vi "Measurement Logic.vi"(8 "error in":errorcluster, 9 "measurement configuration":T2={"Automation Test"=FALSE, "Power sequencing file path"="", "RFSG name"="5842_0", "RFSG port"="", "RFSG attenuation mode"=enum."Constant Attenuation", "RFSG external attenuation (dB)"=2.0, "RFSG s-parameters orientation"=enum."Port2 Towards DUT", "RFSG s2p file path"="", "RFmx name"="5842_0", "RFmx port"="", "RFmx attenuation mode"=enum."Constant Attenuation", "RFmx external attenuation (dB)"=1.2, "RFmx s-parameters orientation"=enum."Port2 Towards DUT", "RFmx s2p file path"="", "RFmx Reference Level (dBm)"=10.0, "RFSG Generation IQ Rate (S/s)"=1250000000.0, "Target Pout Per Tone (dBm)"=10.0, "Start Pin Per Tone (dBm)"=10.0, "Start Center Frequency (Hz)"=10.0, "Start Tone Spacing (Hz)"=10.0, "IM_Sweep Mode"=enum."Power", "Sweep Delay (ms)"=10, "Power Sweep End"=10.0, "Power Sweep Step"=10.0, "Frequency Sweep End"=-4.0, "Frequency Sweep Step"=1.0, "Tone Spacing Sweep End"=-4.0, "Tone Spacing Sweep Step"=1.0} {"Tone Spacing Sweep Step" format="%#.pHz"; "Tone Spacing Sweep End" format="%#.pHz"; "Frequency Sweep Step" format="%#.pHz"; "Frequency Sweep End" format="%#.pHz"; "Power Sweep End" format="%#.6f"; "Sweep Delay (ms)" format="%#_6p"; "Start Tone Spacing (Hz)" format="%#.6p"; "Start Center Frequency (Hz)" format="%#.6p"; "Start Pin Per Tone (dBm)" format="%#.6p"; "Target Pout Per Tone (dBm)" format="%#.6f"; "RFSG Generation IQ Rate (S/s)" format="%#.6f"; "RFmx Reference Level (dBm)" format="%#_6p"; "RFmx external attenuation (dB)" format="%.2f"; "RFSG external attenuation (dB)" format="%.2f"}, 10 "measure call context in":refnum<class "Measure Call Context.lvclass">) -> (0 "error out":errorcluster, 1 "measurement results":T1, 2 "measure call context out":refnum<class "Measure Call Context.lvclass">)   [LabVIEW 2023, in "FPT Intermodulation.lvclass"]
doc: "Contains the core logic for executing the measurement."
uses:
  FPT Intermodulation.lvclass
  <vilib>/Plug-In SDKs/Measurements/Measure Call Context/Measure Call Context.lvclass
  Measurement Configuration.ctl
  Measurement Results.ctl
  <extravilib>/ChannelInstances/Event Messenger-bool/Instantiate.vi
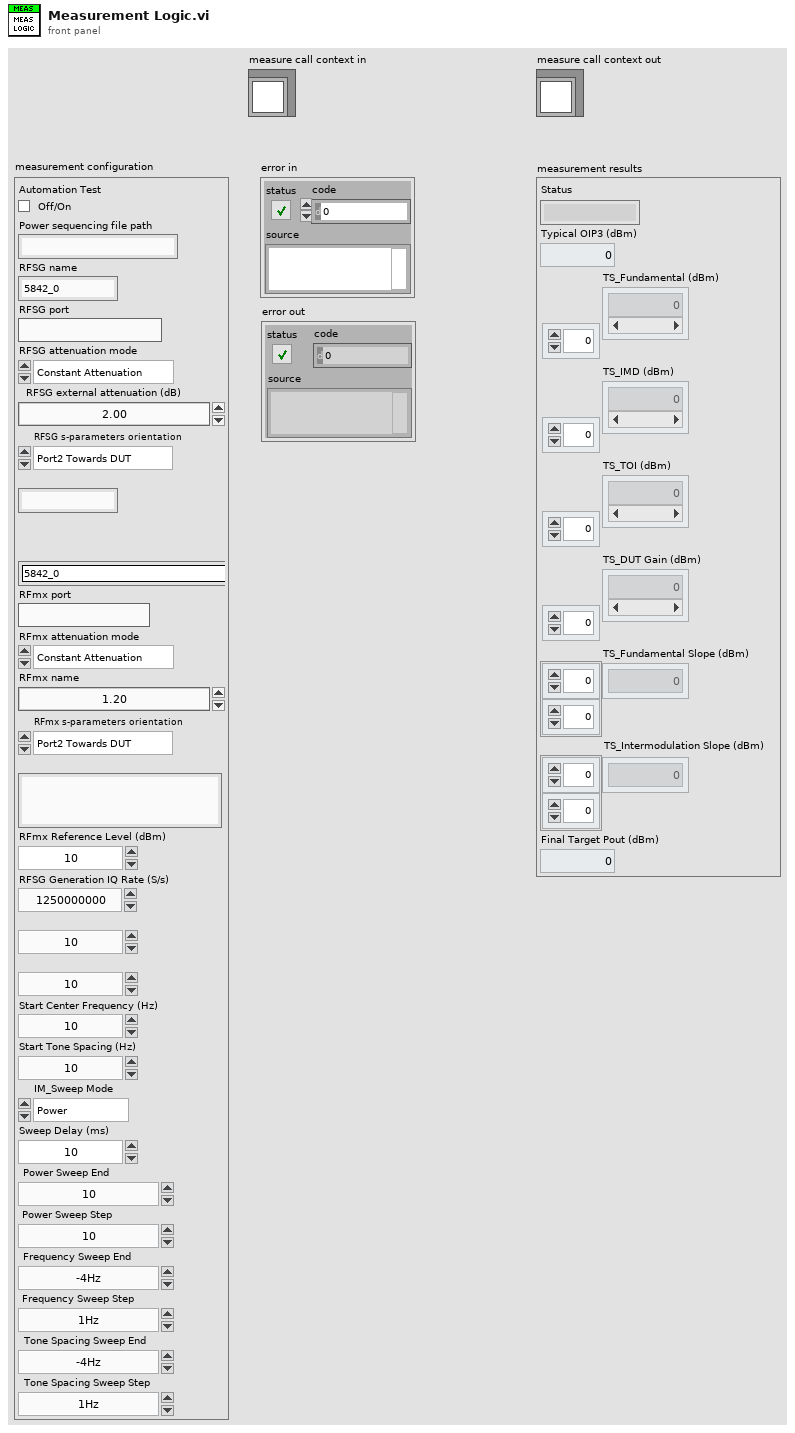
[diagram p1: front panel]
types:
  T1 = typedef "FPT Intermodulation.lvclass/Measurement Results.ctl" = cluster{"Status":string, "Typical OIP3 (dBm)":dbl, "TS_Fundamental (dBm)":dbl[][], "TS_IMD (dBm)":dbl[][], "TS_TOI (dBm)":dbl[][], "TS_DUT Gain (dBm)":dbl[][], "TS_Fundamental Slope (dBm)":dbl[][], "TS_Intermodulation Slope (dBm)":dbl[][], "Final Target Pout (dBm)":dbl}
  T2 = typedef "FPT Intermodulation.lvclass/Measurement Configuration.ctl" = cluster{"Automation Test":bool, "Power sequencing file path":string, "RFSG name":string, "RFSG port":string, "RFSG attenuation mode":enum32{"<None>", "Constant Attenuation", "s2p File"}, "RFSG external attenuation (dB)":dbl, "RFSG s-parameters orientation":enum32{"Port1 Towards DUT", "Port2 Towards DUT"}, "RFSG s2p file path":string, "RFmx name":string, "RFmx port":string, "RFmx attenuation mode":enum32{"<None>", "Constant Attenuation", "s2p File"}, "RFmx external attenuation (dB)":dbl, "RFmx s-parameters orientation":enum32{"Port1 Towards DUT", "Port2 Towards DUT"}, "RFmx s2p file path":string, "RFmx Reference Level (dBm)":dbl, "RFSG Generation IQ Rate (S/s)":dbl, "Target Pout Per Tone (dBm)":dbl, "Start Pin Per Tone (dBm)":dbl, "Start Center Frequency (Hz)":dbl, "Start Tone Spacing (Hz)":dbl, "IM_Sweep Mode":enum32{"Power", "Frequency", "Tone Spacing"}, "Sweep Delay (ms)":u32, "Power Sweep End":dbl, "Power Sweep Step":dbl, "Frequency Sweep End":dbl, "Frequency Sweep Step":dbl, "Tone Spacing Sweep End":dbl, "Tone Spacing Sweep Step":dbl}
  T3 = enum32{"Power On Dut", "De-embedding + Measurement", "Power Off Dut"}[]
  T4 = cluster{"measurement configuration":T2, "measurement results":T1}
  T5 = typedef "RFmx Config - TOI.ctl" = cluster{"Reference Level (dBm)":dbl, "Attenuation":T6}
  T6 = typedef "RFmx Config.ctl" = cluster{"RFmx Name":refnum<k15>, "RFmx Port":string, "Attenuation":cluster{"Mode":enum32{"<None>", "Constant Attenuation", "s2p File"}, "Constant Attenuation":cluster{"RFmx External Attenuation (dB)":dbl}, "s2p File":cluster{"RFmx S-Parameters Orientation":i32, "RFmx Attenuation s2p Path Name":string, "RFmx Attenuation s2p File":path}}}
  T7 = typedef "RFSG Config - TOI.ctl" = cluster{"IQ Rate (S/sec)":dbl, "Number of Samples":i32, "Attenuation":T8}
  T8 = typedef "RFsg Config.ctl" = cluster{"RFSG Name":refnum<k15>, "RFSG Port":string, "Attenuation":cluster{"Mode":enum32{"<None>", "Constant Attenuation", "s2p File"}, "Contant Attenuation":cluster{"RFSG External Attenuation (dB)":dbl}, "s2p File":cluster{"RFSG S-parameters Orientation":i32, "RFSG Attenuation s2p Path Name":string, "RFSG s2p File Path":path}}}
  T9 = typedef "Test Config - TOI.ctl" = cluster{"Target Pout Per Tone (dBm)":dbl, "Start Value":cluster{"Power Level per Tone (dBm)":dbl, "Center Frequency (Hz)":dbl, "Tone Spacing (Hz)":dbl}, "Sweep Settings":cluster{"Mode":enum16{"Power", "Frequency", "Tone Spacing"}, "Sweep Delay (ms)":u32, "Power Sweep End":dbl, "Power Sweep Step":dbl, "Frequency Sweep End":dbl, "Frequency Sweep Step":dbl, "Tone Spacing Sweep End":dbl, "Tone Spacing Sweep Step":dbl}}
  T10 = typedef "Target Pout per Tone Results Cluster - TOI.ctl" = cluster{"Target Pout per Tone (dBm)":dbl, "OIP3 (dBm)":dbl, "IIP3 (dBm)":dbl, "Pin per Tone (dBm)":dbl, "IMD (dBm)":dbl}
  T11 = typedef "Event Messenger-bool.lvlib/))Channel.ctl" = refnum<queue>
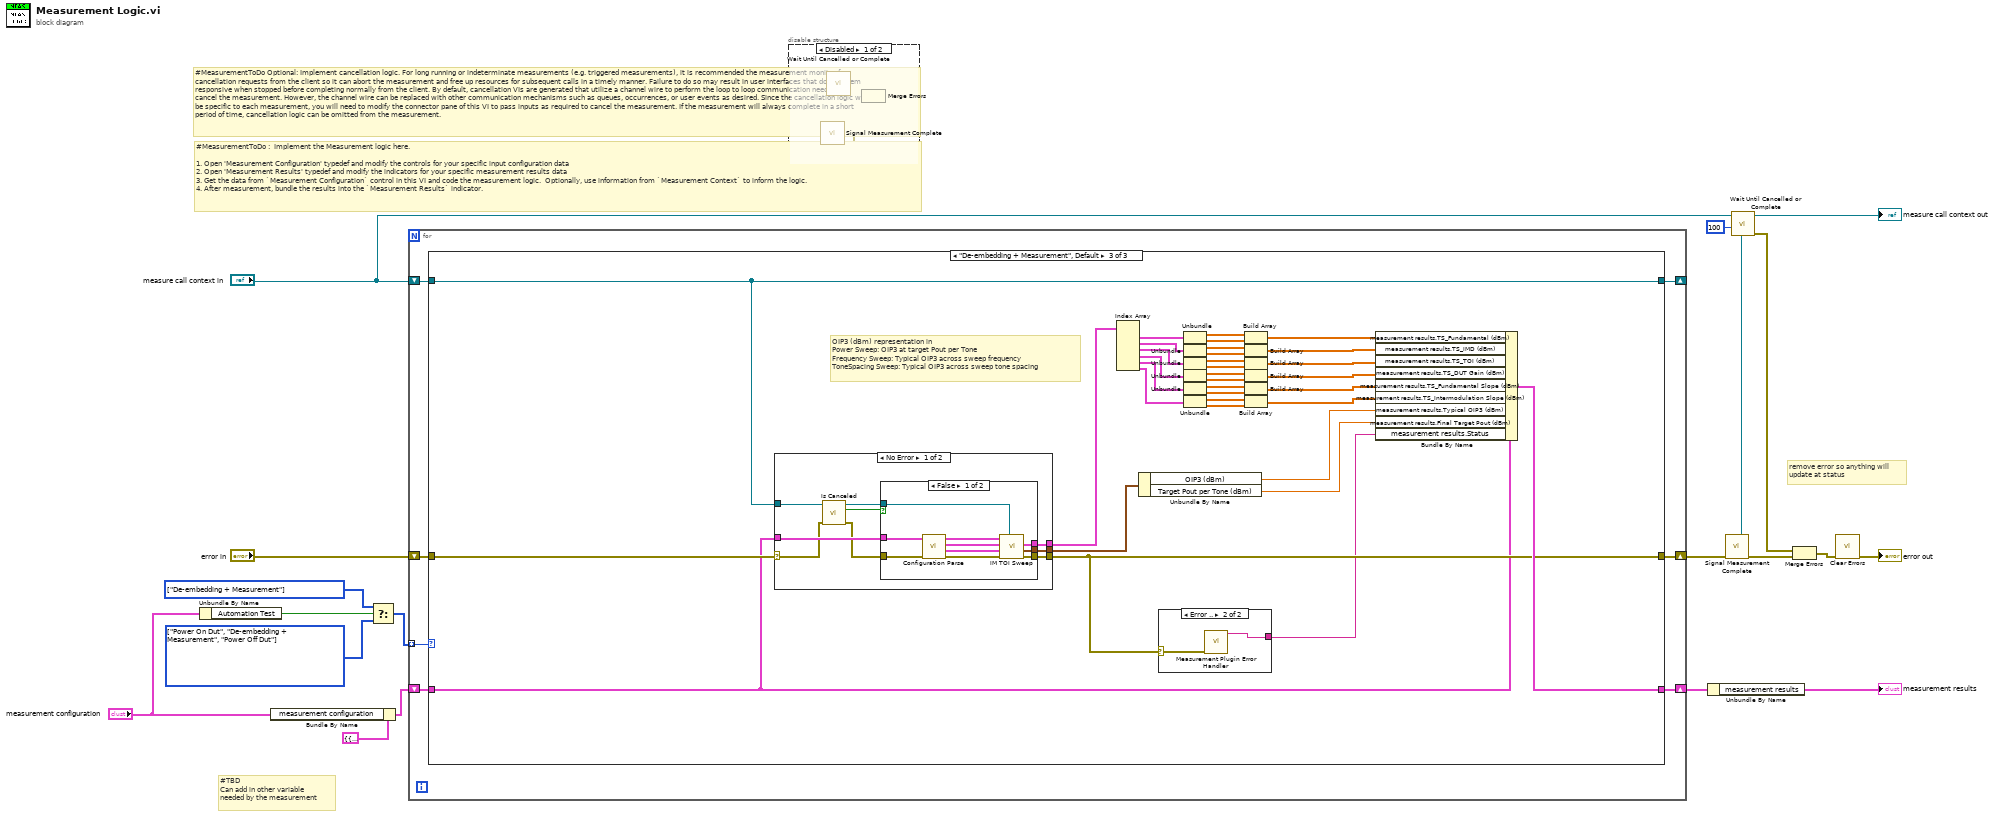
[diagram p0: block diagram]
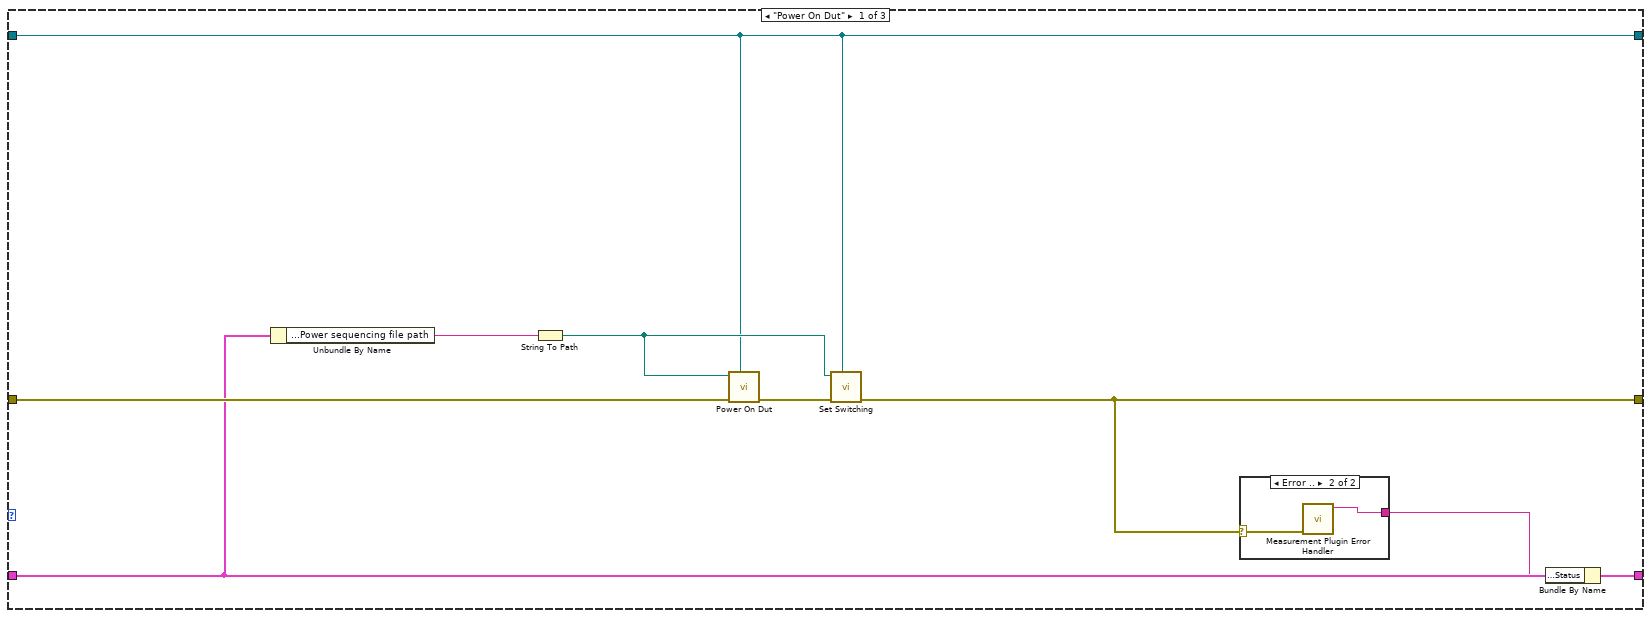
[diagram p2: hidden frame]
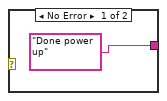
[diagram p3: hidden frame]
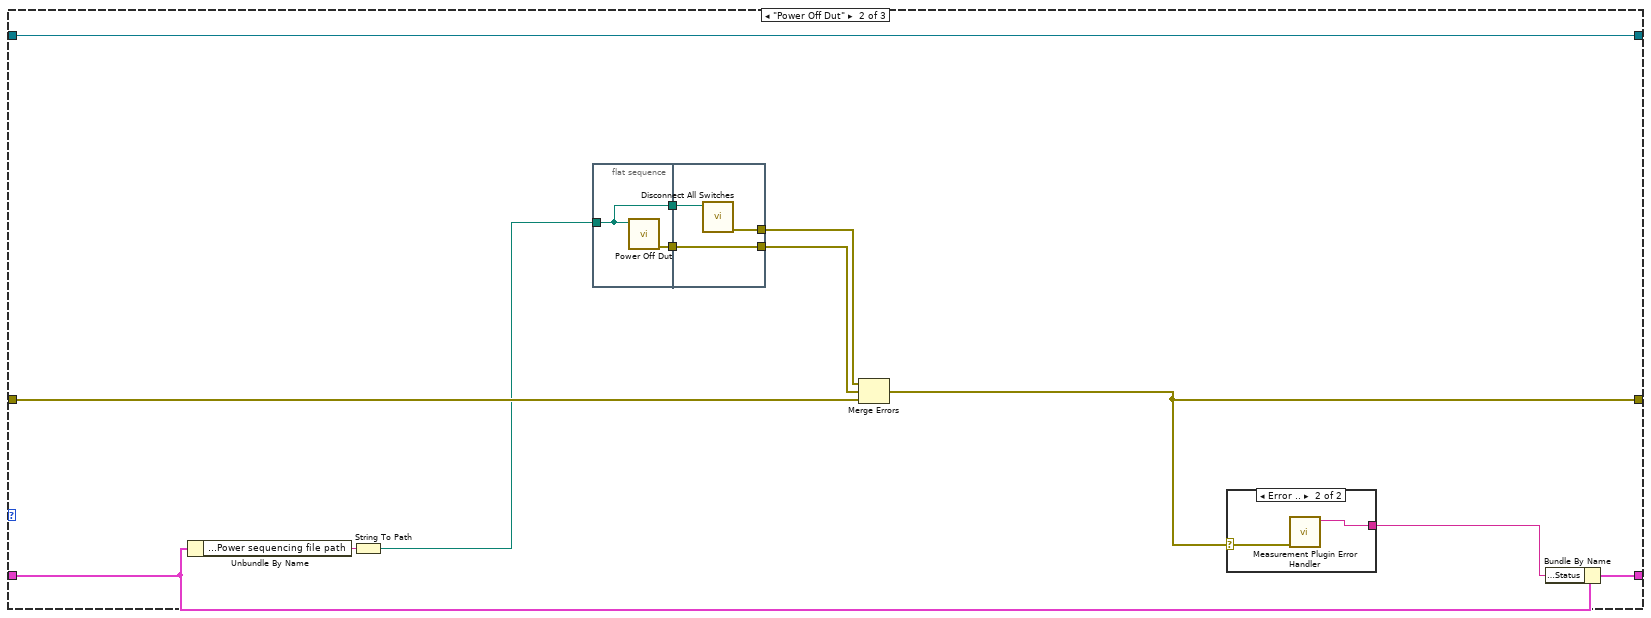
[diagram p4: hidden frame]
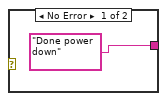
[diagram p5: hidden frame]
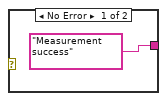
[diagram p6: hidden frame]
diagram:
  w9 = T3 [enum."De-embedding + Measurement"] items=["Power On Dut", "De-embedding + Measurement", "Power Off Dut"]
  w13 = T3 [enum."Power On Dut", enum."De-embedding + Measurement", enum."Power Off Dut"] items=["Power On Dut", "De-embedding + Measurement", "Power Off Dut"]
  # "remove error so anything will\nupdate at status"
  # "#TBD\nCan add in other variable\nneeded by the measurement"
  # "#MeasurementToDo Optional: Implement cancellation logic. For long running or indeterminate measurements (e.g. triggered measurements), it is recommended the measurement monitor for cancellation requests from the client so it can abort the measurement and free up resources for subsequent calls in a timely manner. Failure to do so may result in user interfaces that do not seem responsive when stopped before completing normally from the client. By default, cancellation VIs are generated that utilize a channel wire to perform the loop to loop communication needed to cancel the measurement. However, the channel wire can be replaced with other communication mechanisms such as queues, occurrences, or user events as desired. Since the cancellation logic will be specific to each measurement, you will need to modify the connector pane of this VI to pass inputs as required to cancel the measurement. If the measurement will always complete in a short period of time, cancellation logic can be omitted from the measurement."
  # "#MeasurementToDo :  Implement the Measurement logic here.\n\n1. Open 'Measurement Configuration' typedef and modify the controls for your specific input configuration data\n2. Open 'Measurement Results' typedef and modify the indicators for your specific measurement results data\n3. Get the data from `Measurement Configuration` control in this VI and code the measurement logic.  Optionally, use information from `Measurement Context` to inform the logic.\n4. After measurement, bundle the results into the `Measurement Results` indicator."
  n1 = Unbundle By Name("measurement configuration") -> ("Automation Test"=w10:bool)
  n2 = Bundle By Name(cluster=T4 {"measurement configuration"={"Automation Test"=FALSE, "Power sequencing file path"="", "RFSG name"="5842_0", "RFSG port"="", "RFSG attenuation mode"=enum."Constant Attenuation", "RFSG external attenuation (dB)"=2.0, "RFSG s-parameters orientation"=enum."Port2 Towards DUT", "RFSG s2p file path"="", "RFmx name"="5842_0", "RFmx port"="", "RFmx attenuation mode"=enum."Constant Attenuation", "RFmx external attenuation (dB)"=1.2, "RFmx s-parameters orientation"=enum."Port2 Towards DUT", "RFmx s2p file path"="", "RFmx Reference Level (dBm)"=10.0, "RFSG Generation IQ Rate (S/s)"=1250000000.0, "Target Pout Per Tone (dBm)"=10.0, "Start Pin Per Tone (dBm)"=10.0, "Start Center Frequency (Hz)"=10.0, "Start Tone Spacing (Hz)"=10.0, "IM_Sweep Mode"=enum."Power", "Sweep Delay (ms)"=10, "Power Sweep End"=10.0, "Power Sweep Step"=10.0, "Frequency Sweep End"=-4.0, "Frequency Sweep Step"=1.0, "Tone Spacing Sweep End"=-4.0, "Tone Spacing Sweep Step"=1.0}, "measurement results"={"Status"="", "Typical OIP3 (dBm)"=0.0, "TS_Fundamental (dBm)"=[], "TS_IMD (dBm)"=[], "TS_TOI (dBm)"=[], "TS_DUT Gain (dBm)"=[], "TS_Fundamental Slope (dBm)"=[], "TS_Intermodulation Slope (dBm)"=[], "Final Target Pout (dBm)"=0.0}}, "measurement configuration"="measurement configuration") -> (w17:T4)
  n3 = Select(t=w9, s=w10, f=w13) -> (s? t:f=w12:T3)
  n4 = for {
    tunnel: w12 -> [w25] mode=indexing
    shift-right: [w20] -> w8
    shift-left: "error in" -> [w26]
    shift-right: [w21] -> w16
    shift-left: w17 -> [w24]
    shift-right: [w22] -> _
    shift-left: "measure call context in" -> [w23]
    n5 = case shown="\"De-embedding + Measurement\", Default" w25 {
      tunnel: w26 -> [w35 w45 w71]
      tunnel: w24 -> [w34 w46 w70]
      tunnel: w23 -> [w27 w49 w59]
      tunnel: [w29 w44 w91] -> w20
      tunnel: [w27 w49 w59] -> w22
      tunnel: [w32 w47 w92] -> w21
      frame "Power On Dut" {
        n6 = Unbundle By Name(w34) -> ("measurement configuration.Power sequencing file path"=w31:string)
        n7 = String To Path(string=w31) -> (path=w28:path)
        n8 = call "Power On Dut.vi"("measure call context in"=w27, "error in"=w35, "Power sequencing file path"=w28) -> ("error out"=w30:errorcluster)  [unwired: 7 in, 1 out]
        n9 = call "Set Switching.vi"("measure call context in"=w27, "error in"=w30, "File Path"=w28) -> ("error out"=w29:errorcluster)  [unwired: 7 in, 1 out]
        n10 = case shown="Error .." w29 {
          selector: w29 -> [_ w38]
          tunnel: ["Done power up" w37] -> w33
          frame No Error {
          }
          frame Error {
            n11 = call "Measurement Plugin Error Handler.vi"("error in"=w38) -> ("Status Message (Error)"=w37:string)  [unwired: 9 in, 1 out]
          }
        }
        n12 = Bundle By Name(cluster=w34, "measurement results.Status"=w33) -> (w32:T4)
      }
      frame "Power Off Dut" {
        n13 = Unbundle By Name(w46) -> ("measurement configuration.Power sequencing file path"=w50:string)
        n14 = String To Path(string=w50) -> (path=w41:path)
        n15 = flat-sequence {
          tunnel: w41 -> [w54]
          tunnel: [w55] -> w43
          tunnel: [w54] -> w42
          tunnel: [w58] -> w39
          tunnel: w43 -> [w58]
          tunnel: [w57] -> w40
          tunnel: w42 -> [w56]
          frame #0 {
            n16 = call "Power Off Dut.vi"("Power Sequencing File Path"=w54) -> ("error out"=w55:errorcluster)  [unwired: 10 in]
          }
          frame #1 {
            n17 = call "Disconnect All Switches.vi"("File Path"=w56) -> ("error out"=w57:errorcluster)  [unwired: 10 in]
          }
        }
        n18 = Merge Errors(w40, w39, w45) -> (w44:errorcluster)
        n19 = case shown="Error .." w44 {
          selector: w44 -> [_ w53]
          tunnel: ["Done power down" w52] -> w48
          frame No Error {
          }
          frame Error {
            n20 = call "Measurement Plugin Error Handler.vi"("error in"=w53) -> ("Status Message (Error)"=w52:string)  [unwired: 9 in, 1 out]
          }
        }
        n21 = Bundle By Name(cluster=w46, "measurement results.Status"=w48) -> (w47:T4)
      }
      frame "De-embedding + Measurement", Default {
        # "OIP3 (dBm) representation in\nPower Sweep: OIP3 at target Pout per Tone\nFrequency Sweep: Typical OIP3 across sweep frequency\nToneSpacing Sweep: Typical OIP3 across sweep tone spacing"
        n22 = case shown="No Error" w71 {
          selector: w71 -> [w98 w116]
          tunnel: [w104 w116] -> w91
          tunnel: [w103 _] -> w90
          tunnel: [w102 _] -> w85
          tunnel: w70 -> [w101 _]
          tunnel: w59 -> [w97 _]
          frame No Error {
            n23 = call <vilib>:"Is Canceled.vi"("error in"=w98, "measure call context in"=w97) -> ("error out"=w99:errorcluster, "is canceled?"=w100:bool, "measure call context out"=w96:refnum<class "Measure Call Context.lvclass">)  [unwired: 7 in]
            n24 = case shown="False" w100 {
              tunnel: [w114 w115] -> w104
              tunnel: [w113 _] -> w103
              tunnel: [w112 _] -> w102
              tunnel: w101 -> [w107 _]
              tunnel: w99 -> [w106 w115]
              tunnel: w96 -> [w105 _]
              frame False {
                n25 = call "Configuration Parse.vi"("error in"=w106, "UI Control"=w107) -> ("error out"=w111:errorcluster, "RFmx Settings"=w108:T5, "RFSG Settings"=w109:T7, "Test Configuration"=w110:T9)  [unwired: 6 in]
                n26 = call "IM TOI Sweep.vi"("measure call context in"=w105, "error in"=w111, "RFmx Settings"=w108, "RFSG Settings"=w109, "Test Configuration"=w110) -> ("error out"=w114:errorcluster, "Power Sweep Results - Target Pout per Tone"=w112:T10, "TOI Plot"=w113:cluster{dbl[], dbl[]}[])  [unwired: 2 in, 2 out]
              }
              frame True {
              }
            }
          }
          frame Error {
          }
        }
        n27 = Index Array(array=w90) -> (element #1=w89:cluster{dbl[], dbl[]}, element #2=w88:cluster{dbl[], dbl[]}, element #3=w87:cluster{dbl[], dbl[]}, element #4=w86:cluster{dbl[], dbl[]}, element #5=w63:cluster{dbl[], dbl[]}, element #6=w62:cluster{dbl[], dbl[]})  [unwired: 6 in]
        n28 = Unbundle By Name(w85) -> ("OIP3 (dBm)"=w72:dbl, "Target Pout per Tone (dBm)"=w68:dbl)
        n29 = case shown="Error .." w91 {
          selector: w91 -> [_ w95]
          tunnel: ["Measurement success" w94] -> w69
          frame No Error {
          }
          frame Error {
            n30 = call "Measurement Plugin Error Handler.vi"("error in"=w95) -> ("Status Message (Error)"=w94:string)  [unwired: 9 in, 1 out]
          }
        }
        n31 = Unbundle(w89) -> (w84:dbl[], w83:dbl[])
        n32 = Unbundle(w88) -> (w81:dbl[], w80:dbl[])
        n33 = Unbundle(w87) -> (w78:dbl[], w77:dbl[])
        n34 = Unbundle(w86) -> (w74:dbl[], w75:dbl[])
        n35 = Unbundle(w63) -> (w67:dbl[], w66:dbl[])
        n36 = Unbundle(w62) -> (w65:dbl[], w64:dbl[])
        n37 = Build Array(w84, w83) -> (w82:dbl[][])
        n38 = Build Array(w81, w80) -> (w79:dbl[][])
        n39 = Build Array(w78, w77) -> (w76:dbl[][])
        n40 = Build Array(w74, w75) -> (w73:dbl[][])
        n41 = Build Array(w67, w66) -> (w61:dbl[][])
        n42 = Build Array(w65, w64) -> (w60:dbl[][])
        n43 = Bundle By Name(cluster=w70, "measurement results.TS_Fundamental (dBm)"=w82, "measurement results.TS_IMD (dBm)"=w79, "measurement results.TS_TOI (dBm)"=w76, "measurement results.TS_DUT Gain (dBm)"=w73, "measurement results.TS_Fundamental Slope (dBm)"=w61, "measurement results.TS_Intermodulation Slope (dBm)"=w60, "measurement results.Typical OIP3 (dBm)"=w72, "measurement results.Final Target Pout (dBm)"=w68, "measurement results.Status"=w69) -> (w92:T4)
      }
    }
  }
  n44 = disable-structure shown="Disabled" {
    frame Disabled {
      n45 = call "Signal Measurement Complete.vi"() -> ("error out"=w118:errorcluster, "done channel"=w119:T11)  [unwired: 10 in]
      n46 = call "Wait Until Cancelled or Complete.vi"("done channel"=w119) -> ("error out"=w117:errorcluster)  [unwired: 9 in, 1 out]
      n47 = Merge Errors(w117, w118) -> ()  [unwired: 1 out]
    }
    frame Enabled {
    }
  }
  n48 = Unbundle By Name(w16) -> ("measurement results"=→"measurement results":T1)
  n49 = call "Signal Measurement Complete.vi"("error in (no error)"=w8) -> ("error out"=w7:errorcluster, "done channel"=w5:T11)  [unwired: 9 in]
  n50 = call "Wait Until Cancelled or Complete.vi"("done channel"=w5, "ms polling interval"=100, "measure call context in"="measure call context in") -> ("error out"=w3:errorcluster, "measure call context out"=→"measure call context out":refnum<class "Measure Call Context.lvclass">)  [unwired: 7 in]
  n51 = Merge Errors(w3, w7) -> (w4:errorcluster)
  n52 = call <vilib>:"Clear Errors.vi"("error in (no error)"=w4) -> ("error out"=→"error out":errorcluster)  [unwired: 5 in, 1 out]
